vi "HFRR ADV v016 new software.vi"() -> ()   [LabVIEW 2025] (continued)
        n907 = call "IMAGE ANALYSIS.vi"("Enum"=POST_ANALYSIS_ENUM."SHOW UI", "error in"=w1070) -> ("error out"=w1068:errorcluster)  [unwired: 8 in, 1 out]
        n908 = local write "Zoom Factore"(100.0 ("Zoom Factore")) -> ()
      }
    }
    n909 = case shown="True" w759 {
      selector: w759 -> [_ w1047]
      tunnel: w751 -> [w1044 w1052]
      tunnel: [w1044 w1046] -> _
      frame False {
      }
      frame True {
        n910 = Not(x=w1047) -> (.not. x?=w1045:bool)
        n911 = local read "Zoom Factore"() -> (w1050:dbl)
        n912 = local write "OUT"(w1045) -> ()
        n913 = call "IMAGE ANALYSIS.vi"("Enum"=POST_ANALYSIS_ENUM."ZOOM OUT", "error in"=w1052) -> ("error out"=w1046:errorcluster)  [unwired: 8 in, 1 out]
        n914 = Divide(x=w1050, y=1.2) -> (x/y=w1048:dbl)
        n915 = local write "Zoom Factore"(w1048) -> ()
      }
    }
    n916 = case shown="True" w760 {
      selector: w760 -> [_ w1056]
      tunnel: w751 -> [w1053 w1061]
      tunnel: [w1053 w1054] -> _
      frame False {
      }
      frame True {
        n917 = Not(x=w1056) -> (.not. x?=w1055:bool)
        n918 = local read "Zoom Factore"() -> (w1059:dbl)
        n919 = local write "In"(w1055) -> ()
        n920 = call "IMAGE ANALYSIS.vi"("Enum"=POST_ANALYSIS_ENUM."ZOOM IN", "error in"=w1061) -> ("error out"=w1054:errorcluster)  [unwired: 8 in, 1 out]
        n921 = Multiply(x=w1059, y=1.2) -> (x*y=w1057:dbl)
        n922 = local write "Zoom Factore"(w1057) -> ()
      }
    }
    n923 = case shown="True" w756 {
      selector: w756 -> [_ w1028]
      tunnel: w751 -> [w1026 w1030]
      tunnel: [w1026 w1029] -> _
      frame False {
      }
      frame True {
        n924 = Not(x=w1028) -> (.not. x?=w1027:bool)
        n925 = local write "Clear ROI Tool"(w1027) -> ()
        n926 = call "IMAGE ANALYSIS.vi"("Enum"=POST_ANALYSIS_ENUM."CLEAR ROI", "error in"=w1030) -> ("error out"=w1029:errorcluster)  [unwired: 8 in, 1 out]
      }
    }
    n927 = case shown="True" w758 {
      selector: w758 -> [_ w1040]
      tunnel: w751 -> [w1038 w1043]
      tunnel: [w1038 w1041] -> _
      frame False {
      }
      frame True {
        n928 = Not(x=w1040) -> (.not. x?=w1039:bool)
        n929 = local write "line tool"(w1039) -> ()
        n930 = call "IMAGE ANALYSIS.vi"("Enum"=POST_ANALYSIS_ENUM."DRAW LINE", "error in"=w1043) -> ("error out"=w1041:errorcluster)  [unwired: 8 in, 1 out]
      }
    }
    n931 = case shown="True" w757 {
      selector: w757 -> [_ w1034]
      tunnel: w751 -> [w1032 w1036]
      tunnel: [w1032 w1035] -> _
      frame False {
      }
      frame True {
        n932 = Not(x=w1034) -> (.not. x?=w1033:bool)
        n933 = local write "Rectangle Tool"(w1033) -> ()
        n934 = call "IMAGE ANALYSIS.vi"("Enum"=POST_ANALYSIS_ENUM."DRAW REC", "error in"=w1036) -> ("error out"=w1035:errorcluster)  [unwired: 8 in, 1 out]
      }
    }
    n935 = local read "SCAR MEASURMENT"() -> (w744:enum32{"Auto Scar", "Manual Scar"})
    n936 = local read "Fit to Screen Tool"() -> (w753:bool)
    n937 = local read "Resize Tool"() -> (w752:bool)
    n938 = case shown="\"Manual Scar\", Default" w744 {
      frame "Auto Scar" {
        n939 = property on="Cap Live Image" class="Bool (strict)"("BoolText.Text"="Report" ("Boolean Text.Text")) -> ()  [unwired: 2 in, 2 out]
      }
      frame "Manual Scar", Default {
        n940 = property on="Cap Live Image" class="Bool (strict)"("BoolText.Text"="Save Image" ("Boolean Text.Text")) -> ()  [unwired: 2 in, 2 out]
      }
    }
    n941 = local read "ROI Color Tool"() -> (w754:bool)
    n942 = local read "Pan Tool"() -> (w755:bool)
    n943 = case shown="True" w755 {
      selector: w755 -> [_ w1022]
      tunnel: w751 -> [w1020 w1024]
      tunnel: [w1020 w1023] -> _
      frame False {
      }
      frame True {
        n944 = Not(x=w1022) -> (.not. x?=w1021:bool)
        n945 = call "IMAGE ANALYSIS.vi"("Enum"=POST_ANALYSIS_ENUM."PAN", "error in"=w1024) -> ("error out"=w1023:errorcluster)  [unwired: 8 in, 1 out]
        n946 = local write "Pan Tool"(w1021) -> ()
      }
    }
    n947 = case shown="True" w752 {
      selector: w752 -> [_ w1006]
      tunnel: w751 -> [w1001 w1003]
      tunnel: [w1001 w1002] -> _
      frame False {
      }
      frame True {
        n948 = Not(x=w1006) -> (.not. x?=w1005:bool)
        n949 = local write "Resize Tool"(w1005) -> ()
        n950 = call "IMAGE ANALYSIS.vi"("Enum"=POST_ANALYSIS_ENUM."RESIZE MODE", "error in"=w1003) -> ("error out"=w1002:errorcluster)  [unwired: 8 in, 1 out]
      }
    }
    n951 = case shown="True" w753 {
      selector: w753 -> [_ w1011]
      tunnel: [w1007 w1012] -> _
      tunnel: w751 -> [w1007 w1010]
      frame False {
      }
      frame True {
        n952 = Not(x=w1011) -> (.not. x?=w1009:bool)
        n953 = local write "Zoom Factore"(100.0 ("Zoom Factore")) -> ()
        n954 = local write "Fit to Screen Tool"(w1009) -> ()
        n955 = call "IMAGE ANALYSIS.vi"("Enum"=POST_ANALYSIS_ENUM."FIT", "error in"=w1010) -> ("error out"=w1012:errorcluster)  [unwired: 8 in, 1 out]
      }
    }
    n956 = case shown="True" w754 {
      selector: w754 -> [_ w1017]
      tunnel: [w1014 w1018] -> _
      tunnel: w751 -> [w1014 w1015]
      frame False {
      }
      frame True {
        n957 = Not(x=w1017) -> (.not. x?=w1016:bool)
        n958 = local write "ROI Color Tool"(w1016) -> ()
        n959 = call "IMAGE ANALYSIS.vi"("Enum"=POST_ANALYSIS_ENUM."SET ROI COLOR", "error in"=w1015) -> ("error out"=w1018:errorcluster)  [unwired: 8 in, 1 out]
      }
    }
    n960 = local read "Quit"() -> (w768:bool)
  }
  n961 = while {
    stop <- w1102 stop-if-true
    n962 = local read "Image Path"() -> (w1105:path)
    n963 = local read "Print 3"() -> (w1108:bool)
    n964 = Equal?(x=w1105, y=path "") -> (x = y?=w1104:bool)
    n965 = Not(x=w1104) -> (.not. x?=w1103:bool)
    n966 = property on="Print 3" class="Bool (strict)"("Visible"=w1103) -> ()  [unwired: 2 in, 2 out]
    n967 = case shown="True" w1108 {
      frame False {
        n968 = local write "Rd"(TRUE ("Boolean 7")) -> ()
      }
      frame True {
        n969 = flat-sequence {
          tunnel: [w1148] -> w1116
          tunnel: [w1135] -> w1114
          tunnel: [w1145] -> w1110
          tunnel: w1116 -> [w1157]
          tunnel: [w1157] -> w1115
          tunnel: w1114 -> [w1156]
          tunnel: [w1156] -> w1113
          tunnel: [w1154] -> w1112
          tunnel: [w1153] -> w1111
          tunnel: w1110 -> [w1153]
          tunnel: w1115 -> [w1159]
          tunnel: w1113 -> [w1160]
          tunnel: w1112 -> [_]
          tunnel: w1111 -> [w1158]
          frame #0 {
            n970 = case shown="True" "Rd" {
              frame False {
              }
              frame True {
                n971 = while {
                  tunnel: "abcdefABCDEF" ("string 2") -> [w1127]
                  shift-right: [w1125] -> w1119
                  shift-left: "" -> [w1124]
                  i -> [w1134]
                  stop <- w1133 stop-if-true
                  n972 = Random Number (0-1)() -> (number: 0 to 1=w1128:dbl)
                  n973 = Multiply(x=w1128, y=62.0) -> (x*y=w1130:dbl)
                  n974 = Decrement(x="Length 2") -> (x-1=w1123:i16)
                  n975 = To Word Integer(number=w1130) -> (16bit integer=w1131:i16)
                  n976 = String Subset(string=w1127, offset (0)=w1131, length (rest)=1 ("length (rest)")) -> (substring=w1126:string)
                  n977 = Greater Or Equal?(x=w1134, y=w1123) -> (x >= y?=w1133:bool)
                  n978 = Concatenate Strings(w1126, w1124) -> (w1125:string)
                }
                "String 10" <- w1119
                n979 = local write "Rd"(FALSE ("Boolean 7")) -> ()
              }
            }
          }
          frame #1 {
            w1146 = "_resized.jpg" ("command line")
            (unwired) ".jpg -resize 320x240 " ("string")
            (unwired) "Choose an Image File" ("prompt")
            # "-resize 1798x425"
            n980 = local read "Image Path"() -> (w1140:path)
            n981 = Strip Path(path=w1140) -> (stripped path=w1135:path, name=w1136:string)
            n982 = Match Pattern(string=w1136, regular expression=".jpg") -> (before substring=→"before substring 2":string, after substring=→"after substring":string)  [unwired: 1 in, 2 out]
            n983 = Match Pattern(string=w1136, regular expression="\\") -> (before substring=w1142:string)  [unwired: 1 in, 3 out]
            n984 = Match Pattern(string=w1142, regular expression=".jpg") -> (before substring=w1141:string)  [unwired: 1 in, 3 out]
            n985 = Concatenate Strings("cmd /c convert " ("string"), w1141, ".jpg -resize 320x240  " ("command line"), w1141, w1146) -> (w1149:string)
            n986 = call <vilib>:"System Exec.vi"("run minimized? (F)"=TRUE, "wait until completion? (T)"=TRUE, "working directory"=w1135, "command line"=w1149) -> ("error out"=w1148:errorcluster)  [unwired: 4 in, 3 out]
            "error out 2" <- w1148
            n987 = Concatenate Strings(w1141, w1146) -> (w1145:string)
          }
          frame #2 {
            n988 = Wait (ms)(milliseconds to wait=u32 2000 ("millisecond timer value")) -> (millisecond timer value=w1154:u32)
          }
          frame #3 {
            n989 = case shown="No Error" w1159 {
              tunnel: w1160 -> [w1163 _]
              tunnel: w1158 -> [w1161 _]
              frame No Error {
                (unwired) ".jpg" ("string")
                n990 = Path To String(path=w1163) -> (string=w1167:string)
                n991 = Concatenate Strings(w1167, "\\" ("string"), w1161) -> (w1166:string)
                n992 = String To Path(string=w1166) -> (path=w1165:path)
                n993 = call <vilib>:"Read JPEG File.vi"("path to JPEG file"=w1165) -> ("image data"=w1169:T16)  [unwired: 8 in, 2 out]
                "image data" <- w1169
                n994 = local write "Print 3"(FALSE ("Print 2")) -> ()
                n995 = call <vilib>:"Draw Flattened Pixmap.vi"("image data"=w1169) -> ("new picture"=→"new picture":picture)  [unwired: 8 in]
              }
              frame Error {
              }
            }
          }
        }
      }
    }
    n996 = Wait (ms)(milliseconds to wait=u32 20 ("millisecond timer value")) -> ()  [unwired: 1 out]
    n997 = local read "Quit"() -> (w1102:bool)
  }
  n998 = while {
    tunnel: w33 -> [_]
    tunnel: w17 -> [_]
    stop <- w1200 stop-if-true
    # "New Adv Logics"
    n999 = local read "Main Tab"() -> (w1180:T2)
    n1000 = local read "Main Tab"() -> (w1198:T2)
    n1001 = local read "Sign In"() -> (w1197:bool)
    n1002 = case shown="\"Adv Scar\"" w1180 {
      frame "HOME", Default {
        n1003 = local read "LIVE FEED MIN TEMP"() -> (w1333:bool)
        n1004 = local write "LIVE FEED MAX TEMP"(TRUE ("LIVE FEED MAX TEMP")) -> ()
        n1005 = local read "CAMERA ROI MIN TEMP"() -> (w1331:bool)
        n1006 = case shown="True" w1333 {
          selector: w1333 -> [_ w1340]
          frame False {
          }
          frame True {
            n1007 = Not(x=w1340) -> (.not. x?=w1339:bool)
            n1008 = local write "LIVE FEED MIN TEMP"(w1339) -> ()
            n1009 = call "CAMERA LIVE FEED FGV.vi"("Enum - Menu"=CAMERA_LIVE_FEED_ENUM."CAMERA MINIMIZE") -> ()  [unwired: 9 in, 2 out]
          }
        }
        n1010 = case shown="True" w1331 {
          selector: w1331 -> [_ w1337]
          frame False {
          }
          frame True {
            n1011 = Not(x=w1337) -> (.not. x?=w1336:bool)
            n1012 = local write "CAMERA ROI MIN TEMP"(w1336) -> ()
            n1013 = call "IMAGE ANALYSIS.vi"("Enum"=POST_ANALYSIS_ENUM."MINIMIZE UI") -> ()  [unwired: 9 in, 2 out]
          }
        }
        n1014 = local write "CAMERA ROI MAX TEMP"(TRUE ("CAMERA ROI MAX TEMP")) -> ()
      }
      frame "Test Setup" {
        n1015 = local read "LIVE FEED MIN TEMP"() -> (w1343:bool)
        n1016 = local read "CAMERA ROI MIN TEMP"() -> (w1341:bool)
        n1017 = local write "LIVE FEED MAX TEMP"(TRUE ("LIVE FEED MAX TEMP")) -> ()
        n1018 = case shown="True" w1343 {
          selector: w1343 -> [_ w1350]
          frame False {
          }
          frame True {
            n1019 = Not(x=w1350) -> (.not. x?=w1349:bool)
            n1020 = local write "LIVE FEED MIN TEMP"(w1349) -> ()
            n1021 = call "CAMERA LIVE FEED FGV.vi"("Enum - Menu"=CAMERA_LIVE_FEED_ENUM."CAMERA MINIMIZE") -> ()  [unwired: 9 in, 2 out]
          }
        }
        n1022 = case shown="True" w1341 {
          selector: w1341 -> [_ w1347]
          frame False {
          }
          frame True {
            n1023 = Not(x=w1347) -> (.not. x?=w1346:bool)
            n1024 = local write "CAMERA ROI MIN TEMP"(w1346) -> ()
            n1025 = call "IMAGE ANALYSIS.vi"("Enum"=POST_ANALYSIS_ENUM."MINIMIZE UI") -> ()  [unwired: 9 in, 2 out]
          }
        }
        n1026 = local write "CAMERA ROI MAX TEMP"(TRUE ("CAMERA ROI MAX TEMP")) -> ()
      }
      frame "Acquire" {
        n1027 = local read "LIVE FEED MIN TEMP"() -> (w1353:bool)
        n1028 = local write "LIVE FEED MAX TEMP"(TRUE ("LIVE FEED MAX TEMP")) -> ()
        n1029 = local read "CAMERA ROI MIN TEMP"() -> (w1351:bool)
        n1030 = case shown="True" w1353 {
          selector: w1353 -> [_ w1360]
          frame False {
          }
          frame True {
            n1031 = Not(x=w1360) -> (.not. x?=w1359:bool)
            n1032 = local write "LIVE FEED MIN TEMP"(w1359) -> ()
            n1033 = call "CAMERA LIVE FEED FGV.vi"("Enum - Menu"=CAMERA_LIVE_FEED_ENUM."CAMERA MINIMIZE") -> ()  [unwired: 9 in, 2 out]
          }
        }
        n1034 = case shown="True" w1351 {
          selector: w1351 -> [_ w1357]
          frame False {
          }
          frame True {
            n1035 = Not(x=w1357) -> (.not. x?=w1356:bool)
            n1036 = local write "CAMERA ROI MIN TEMP"(w1356) -> ()
            n1037 = call "IMAGE ANALYSIS.vi"("Enum"=POST_ANALYSIS_ENUM."MINIMIZE UI") -> ()  [unwired: 9 in, 2 out]
          }
        }
        n1038 = local write "CAMERA ROI MAX TEMP"(TRUE ("CAMERA ROI MAX TEMP")) -> ()
      }
      frame "Adv Scar" {
        n1039 = local read "CAMERA ROI MIN TEMP"() -> (w1361:bool)
        n1040 = case shown="True" "LIVE FEED MAX TEMP" {
          selector: "LIVE FEED MAX TEMP" -> [_ w1382]
          frame False {
          }
          frame True {
            n1041 = Not(x=w1382) -> (.not. x?=w1381:bool)
            n1042 = local write "LIVE FEED MAX TEMP"(w1381) -> ()
            n1043 = call "CAMERA LIVE FEED FGV.vi"("Enum - Menu"=CAMERA_LIVE_FEED_ENUM."CAMERA RESTORE") -> ("error out"=w1372:errorcluster)  [unwired: 9 in, 1 out]
            n1044 = Type Cast(type=30, x=0) -> (*(type *) &x=w1376:i32)
            n1045 = Add(x=w1376, y=48) -> (x+y=w1377:i32)
            n1046 = call "CAMERA LIVE FEED FGV.vi"("Enum - Menu"=CAMERA_LIVE_FEED_ENUM."CAMERA MODE SET", "error in (no error)"=w1372, "CAMERA MODE"=w1377) -> ("error out"=w1369:errorcluster)  [unwired: 7 in, 1 out]
            n1047 = call "CAMERA LIVE FEED FGV.vi"("Enum - Menu"=CAMERA_LIVE_FEED_ENUM."CAMERA GRAY", "error in (no error)"=w1369) -> ("error out"=w1368:errorcluster)  [unwired: 8 in, 1 out]
            n1048 = call "LIST FILE NAMES.vi"("error in (no error)"=w1368) -> ("error out"=w1378:errorcluster, "filenames"=w1379:string[])  [unwired: 9 in]
            n1049 = property on="FILE 3" class="CmbBox"(error in=w1378, "Strings[]"=w1379) -> ()  [unwired: 1 in, 2 out]
          }
        }
        n1050 = case shown="True" w1361 {
          selector: w1361 -> [_ w1367]
          frame False {
          }
          frame True {
            n1051 = Not(x=w1367) -> (.not. x?=w1366:bool)
            n1052 = local write "CAMERA ROI MIN TEMP"(w1366) -> ()
            n1053 = call "IMAGE ANALYSIS.vi"("Enum"=POST_ANALYSIS_ENUM."MINIMIZE UI") -> ()  [unwired: 9 in, 2 out]
          }
        }
        n1054 = local write "CAMERA ROI MAX TEMP"(TRUE ("CAMERA ROI MAX TEMP")) -> ()
        "LIVE FEED MIN TEMP" <- TRUE ("LIVE FEED MIN TEMP")
      }
      frame "Adv Scar Report" {
        n1055 = local read "CAMERA ROI MAX TEMP"() -> (w1383:bool)
        n1056 = local read "LIVE FEED MIN TEMP"() -> (w1385:bool)
        n1057 = local write "LIVE FEED MAX TEMP"(TRUE ("LIVE FEED MAX TEMP")) -> ()
        n1058 = case shown="True" w1385 {
          selector: w1385 -> [_ w1394]
          frame False {
          }
          frame True {
            n1059 = Not(x=w1394) -> (.not. x?=w1393:bool)
            n1060 = local write "LIVE FEED MIN TEMP"(w1393) -> ()
            n1061 = call "CAMERA LIVE FEED FGV.vi"("Enum - Menu"=CAMERA_LIVE_FEED_ENUM."CAMERA MINIMIZE") -> ()  [unwired: 9 in, 2 out]
          }
        }
        n1062 = case shown="True" w1383 {
          selector: w1383 -> [_ w1391]
          frame False {
          }
          frame True {
            n1063 = Not(x=w1391) -> (.not. x?=w1389:bool)
            n1064 = local write "CAMERA ROI MAX TEMP"(w1389) -> ()
            n1065 = call "IMAGE ANALYSIS.vi"("Enum"=POST_ANALYSIS_ENUM."SHOW UI") -> ("error out"=w1388:errorcluster)  [unwired: 9 in, 1 out]
            n1066 = call "LIST FILE NAMES.vi"("error in (no error)"=w1388) -> ("filenames"=w1387:string[])  [unwired: 9 in, 1 out]
            n1067 = property on="Test File List :" class="CmbBox"("Strings[]"=w1387) -> ()  [unwired: 2 in, 2 out]
          }
        }
        n1068 = local write "CAMERA ROI MIN TEMP"(TRUE ("CAMERA ROI MIN TEMP")) -> ()
      }
      frame "Compare Files" {
        n1069 = local read "LIVE FEED MIN TEMP"() -> (w1397:bool)
        n1070 = local write "LIVE FEED MAX TEMP"(TRUE ("LIVE FEED MAX TEMP")) -> ()
        n1071 = local read "CAMERA ROI MIN TEMP"() -> (w1395:bool)
        n1072 = case shown="True" w1397 {
          selector: w1397 -> [_ w1404]
          frame False {
          }
          frame True {
            n1073 = Not(x=w1404) -> (.not. x?=w1403:bool)
            n1074 = local write "LIVE FEED MIN TEMP"(w1403) -> ()
            n1075 = call "CAMERA LIVE FEED FGV.vi"("Enum - Menu"=CAMERA_LIVE_FEED_ENUM."CAMERA MINIMIZE") -> ()  [unwired: 9 in, 2 out]
          }
        }
        n1076 = case shown="True" w1395 {
          selector: w1395 -> [_ w1401]
          frame False {
          }
          frame True {
            n1077 = Not(x=w1401) -> (.not. x?=w1400:bool)
            n1078 = local write "CAMERA ROI MIN TEMP"(w1400) -> ()
            n1079 = call "IMAGE ANALYSIS.vi"("Enum"=POST_ANALYSIS_ENUM."MINIMIZE UI") -> ()  [unwired: 9 in, 2 out]
          }
        }
        n1080 = local write "CAMERA ROI MAX TEMP"(TRUE ("CAMERA ROI MAX TEMP")) -> ()
      }
      frame "About" {
        n1081 = local read "LIVE FEED MIN TEMP"() -> (w1407:bool)
        n1082 = local write "LIVE FEED MAX TEMP"(TRUE ("LIVE FEED MAX TEMP")) -> ()
        n1083 = local read "CAMERA ROI MIN TEMP"() -> (w1406:bool)
        n1084 = case shown="True" w1407 {
          selector: w1407 -> [_ w1414]
          frame False {
          }
          frame True {
            n1085 = Not(x=w1414) -> (.not. x?=w1413:bool)
            n1086 = local write "LIVE FEED MIN TEMP"(w1413) -> ()
            n1087 = call "CAMERA LIVE FEED FGV.vi"("Enum - Menu"=CAMERA_LIVE_FEED_ENUM."CAMERA MINIMIZE") -> ()  [unwired: 9 in, 2 out]
          }
        }
        n1088 = case shown="True" w1406 {
          selector: w1406 -> [_ w1411]
          frame False {
          }
          frame True {
            n1089 = Not(x=w1411) -> (.not. x?=w1410:bool)
            n1090 = local write "CAMERA ROI MIN TEMP"(w1410) -> ()
            n1091 = call "IMAGE ANALYSIS.vi"("Enum"=POST_ANALYSIS_ENUM."MINIMIZE UI") -> ()  [unwired: 9 in, 2 out]
          }
        }
        n1092 = local write "CAMERA ROI MAX TEMP"(TRUE ("CAMERA ROI MIN TEMP")) -> ()
      }
      frame "Advance" {
        n1093 = local read "LIVE FEED MIN TEMP"() -> (w1417:bool)
        n1094 = local write "LIVE FEED MAX TEMP"(TRUE ("LIVE FEED MAX TEMP")) -> ()
        n1095 = local read "CAMERA ROI MIN TEMP"() -> (w1415:bool)
        n1096 = case shown="True" w1417 {
          selector: w1417 -> [_ w1424]
          frame False {
          }
          frame True {
            n1097 = Not(x=w1424) -> (.not. x?=w1423:bool)
            n1098 = local write "LIVE FEED MIN TEMP"(w1423) -> ()
            n1099 = call "CAMERA LIVE FEED FGV.vi"("Enum - Menu"=CAMERA_LIVE_FEED_ENUM."CAMERA MINIMIZE") -> ()  [unwired: 9 in, 2 out]
          }
        }
        n1100 = local write "CAMERA ROI MAX TEMP"(TRUE ("CAMERA ROI MAX TEMP")) -> ()
        n1101 = case shown="True" w1415 {
          selector: w1415 -> [_ w1421]
          frame False {
          }
          frame True {
            n1102 = Not(x=w1421) -> (.not. x?=w1420:bool)
            n1103 = local write "CAMERA ROI MIN TEMP"(w1420) -> ()
            n1104 = call "IMAGE ANALYSIS.vi"("Enum"=POST_ANALYSIS_ENUM."MINIMIZE UI") -> ()  [unwired: 9 in, 2 out]
          }
        }
      }
      frame "Mooha" {
        n1105 = local read "LIVE FEED MIN TEMP"() -> (w1427:bool)
        n1106 = local write "LIVE FEED MAX TEMP"(TRUE ("LIVE FEED MAX TEMP")) -> ()
        n1107 = local read "CAMERA ROI MIN TEMP"() -> (w1425:bool)
        n1108 = case shown="True" w1427 {
          selector: w1427 -> [_ w1434]
          frame False {
          }
          frame True {
            n1109 = Not(x=w1434) -> (.not. x?=w1433:bool)
            n1110 = local write "LIVE FEED MIN TEMP"(w1433) -> ()
            n1111 = call "CAMERA LIVE FEED FGV.vi"("Enum - Menu"=CAMERA_LIVE_FEED_ENUM."CAMERA MINIMIZE") -> ()  [unwired: 9 in, 2 out]
          }
        }
        n1112 = local write "CAMERA ROI MAX TEMP"(TRUE ("CAMERA ROI MAX TEMP")) -> ()
        n1113 = case shown="True" w1425 {
          selector: w1425 -> [_ w1431]
          frame False {
          }
          frame True {
            n1114 = Not(x=w1431) -> (.not. x?=w1430:bool)
            n1115 = local write "CAMERA ROI MIN TEMP"(w1430) -> ()
            n1116 = call "IMAGE ANALYSIS.vi"("Enum"=POST_ANALYSIS_ENUM."MINIMIZE UI") -> ()  [unwired: 9 in, 2 out]
          }
        }
      }
    }
    n1117 = local read "Auto Start Test"() -> (w1171:bool)
    n1118 = case shown="True" "sign in temp" {
      frame False {
      }
      frame True {
        w1207 = 1 ("y")
        n1119 = local read "USERNAME"() -> (w1213:string)
        n1120 = local read "USER ID"() -> (w1210:string)
        n1121 = call <vilib>:"Trim Whitespace.vi"("string"=w1213) -> ("trimmed string"=w1212:string)  [unwired: 1 in]
        n1122 = call <vilib>:"Trim Whitespace.vi"("string"=w1210) -> ("trimmed string"=w1211:string)  [unwired: 1 in]
        n1123 = String Length(string=w1212) -> (length=w1209:i32)
        n1124 = String Length(string=w1211) -> (length=w1208:i32)
        n1125 = Greater?(x=w1209, y=w1207) -> (0:w1206:bool)
        n1126 = Greater?(x=w1208, y=w1207) -> (0:w1205:bool)
        n1127 = And(x=w1206, y=w1205) -> (x .and. y?=w1204:bool)
        n1128 = case shown="True" w1204 {
          frame False {
            n1129 = property on="Sign In" class="Bool (strict)"("DisabledEnum"=T18."Disabled" ("Disabled")) -> ()  [unwired: 2 in, 2 out]
          }
          frame True {
            n1130 = property on="Sign In" class="Bool (strict)"("DisabledEnum"=T18."Enabled" ("Disabled")) -> ()  [unwired: 2 in, 2 out]
          }
        }
      }
    }
    n1131 = local read "Air Temperature"() -> (w1188:bool)
    n1132 = local read "Coefficient Of Friction"() -> (w1189:bool)
    n1133 = case shown="False" w1171 {
      frame False {
        n1134 = local read "Auto stop temp"() -> (w1201:bool)
        n1135 = case shown="True" w1201 {
          frame False {
          }
          frame True {
            n1136 = local write "Auto Start Temp"(FALSE ("Auto Start Temp")) -> ()
          }
        }
      }
      frame True {
        "Auto stop temp" <- TRUE ("Auto stop temp")
      }
    }
    n1137 = local read "Humidity"() -> (w1187:bool)
    n1138 = case shown="\"HOME\"" w1198 {
      frame "HOME" {
        n1139 = local write "main tab sub"(enum32{"Page 1", "Page 2"}."Page 1" ("main tab sub")) -> ()
      }
      frame Default {
        n1140 = local write "main tab sub"(enum32{"Page 1", "Page 2"}."Page 2" ("main tab sub")) -> ()
      }
    }
    n1141 = case shown="True" w1197 {
      selector: w1197 -> [_ w1548]
      frame False {
      }
      frame True {
        n1142 = Not(x=w1548) -> (.not. x?=w1547:bool)
        n1143 = local write "Sign In"(w1547) -> ()
        n1144 = local write "Main Dashboard Buttons"(T24."Test Setup" ("Main Dashboard Buttons")) -> ()
      }
    }
    n1145 = case shown="\"Numeric Display\", Default" "Num/Graph" {
      frame "Numeric Display", Default {
        n1146 = property on="Single/Multiple" class="RadioBtnsControl (strict)"("Visible"=FALSE) -> ()  [unwired: 2 in, 2 out]
        n1147 = property on="Single - Graph" class="Ring (strict)"("Visible"=FALSE) -> ()  [unwired: 2 in, 2 out]
        n1148 = local write "Main Tab Display"(T4."Dashboard 1" ("Main Tab Display")) -> ()
      }
      frame "Graph Display" {
        n1149 = property on="Single/Multiple" class="RadioBtnsControl (strict)"("Visible"=TRUE) -> ()  [unwired: 2 in, 2 out]
        n1150 = case shown="\"Multiple\"" "Single/Multiple" {
          frame "Single ", Default {
            n1151 = property on="Single - Graph" class="Ring (strict)"("Visible"=TRUE) -> ()  [unwired: 2 in, 2 out]
            n1152 = local write "Main Tab Display"(T4."Dashboard 3" ("Main Tab Display")) -> ()
          }
          frame "Multiple" {
            n1153 = property on="Single - Graph" class="Ring (strict)"("Visible"=FALSE) -> ()  [unwired: 2 in, 2 out]
            n1154 = local write "Main Tab Display"(T4."Dashboard 2" ("Main Tab Display")) -> ()
          }
        }
      }
    }
    n1155 = local read "Stroke"() -> (w1186:bool)
    n1156 = local read "USERNAME"() -> (w1192:string)
    n1157 = local read "USER ID"() -> (w1191:string)
    n1158 = case shown="True" w1189 {
      selector: w1189 -> [_ w1474]
      frame False {
      }
      frame True {
        n1159 = Not(x=w1474) -> (.not. x?=w1473:bool)
        n1160 = local write "Coefficient Of Friction"(w1473) -> ()
        n1161 = local write "Tab Control 2"(T6."Coefficient Of Friction" ("Tab Control 2")) -> ()
      }
    }
    n1162 = case shown="True" w1188 {
      selector: w1188 -> [_ w1471]
      frame False {
      }
      frame True {
        n1163 = Not(x=w1471) -> (.not. x?=w1469:bool)
        n1164 = local write "Air Temperature"(w1469) -> ()
        n1165 = local write "Tab Control 2"(T6."Air Temperature" ("Tab Control 2")) -> ()
      }
    }
    n1166 = local write "Operator ID"(w1191) -> ()
    n1167 = case shown="True" w1186 {
      selector: w1186 -> [_ w1465]
      frame False {
      }
      frame True {
        n1168 = Not(x=w1465) -> (.not. x?=w1463:bool)
        n1169 = local write "Stroke"(w1463) -> ()
        n1170 = local write "Tab Control 2"(T6."Stroke" ("Tab Control 2")) -> ()
      }
    }
    n1171 = local write "tested by"(w1192) -> ()
    n1172 = case shown="True" w1187 {
      selector: w1187 -> [_ w1468]
      frame False {
      }
      frame True {
        n1173 = Not(x=w1468) -> (.not. x?=w1466:bool)
        n1174 = local write "Humidity"(w1466) -> ()
        n1175 = local write "Tab Control 2"(T6."Humidity" ("Tab Control 2")) -> ()
      }
    }
    n1176 = case shown="\"Calibration\"" "Main Dashboard Buttons" {
      tunnel: [T2."HOME" ("Main Tab") T2."Test Setup" ("Main Tab") T2."Acquire" ("Main Tab") T2."Adv Scar" ("Main Tab") T2."Adv Scar Report" ("Main Tab") T2."Compare Files" ("Main Tab") T2."Calibration" ("Main Tab") T2."About" ("Main Tab") T2."Advance" ("Main Tab")] -> w1170
      frame "Home", Default {
      }
      frame "Test Setup" {
      }
      frame "Dashboard" {
      }
      frame "Imaging" {
      }
      frame "Report" {
      }
      frame "Analysis" {
      }
      frame "Calibration" {
      }
      frame "About" {
      }
      frame "Advance" {
      }
    }
    n1177 = Wait (ms)(milliseconds to wait=u32 100) -> ()  [unwired: 1 out]
    n1178 = local read "Main Tab Display"() -> (w1190:T4)
    n1179 = local write "Main Tab"(w1170) -> ()
    n1180 = case shown="\"Dashboard 3\"" w1190 {
      frame "Dashboard 1", Default {
        n1181 = property on="Reset Graph" class="Bool (strict)"("Visible"=FALSE) -> ()  [unwired: 2 in, 2 out]
      }
      frame "Dashboard 2" {
        n1182 = property on="Reset Graph" class="Bool (strict)"("Visible"=TRUE) -> ()  [unwired: 2 in, 2 out]
      }
      frame "Dashboard 3" {
        n1183 = property on="Reset Graph" class="Bool (strict)"("Visible"=TRUE) -> ()  [unwired: 2 in, 2 out]
      }
    }
    n1184 = local read "SCAR MEASURMENT"() -> (w1178:enum32{"Auto Scar", "Manual Scar"})
    n1185 = local read "Humidity"() -> (w1193:bool)
    n1186 = local read "Cap Live Image"() -> (w1175:bool)
    n1187 = local read "Sample Temperature"() -> (w1185:bool)
    n1188 = local read "Air Temp vs Humidity"() -> (w1183:bool)
    n1189 = local read "Frequency"() -> (w1184:bool)
    n1190 = case shown="True" w1193 {
      frame False {
        n1191 = local write "Humidity On Command"(TRUE ("Humidity On Command")) -> ()
        n1192 = case shown="True" "Humidity Off Command" {
          selector: "Humidity Off Command" -> [_ w1481]
          frame False {
          }
          frame True {
            n1193 = stacked-sequence {
              frame #0 {
                n1194 = local read "WriteHumidity"() -> (w1483:string[])
                n1195 = Insert Into Array(array=w1483, new element="R;1" ("new element/subarray")) -> (w1484:string[])  [unwired: 1 in]
                n1196 = local write "WriteHumidity"(w1484) -> ()
              }
              frame #1 {
                n1197 = Wait (ms)(milliseconds to wait=u32 2000) -> ()  [unwired: 1 out]
              }
              frame #2 {
                n1198 = local read "EVENT LOG"() -> (w1490:string)
                n1199 = local read "WriteHumidity"() -> (w1487:string[])
                n1200 = call "Event Log.vi"("Content"="Humidity Control Off" ("string"), "EVENT LOG"=w1490) -> ("EVENT LOG"=w1491:string)  [unwired: 8 in, 1 out]
                n1201 = local write "EVENT LOG"(w1491) -> ()
                n1202 = Insert Into Array(array=w1487, new element="R;1" ("new element/subarray")) -> (w1488:string[])  [unwired: 1 in]
                n1203 = local write "WriteHumidity"(w1488) -> ()
              }
            }
            n1204 = Not(x=w1481) -> (.not. x?=w1480:bool)
            n1205 = local write "Humidity Off Command"(w1480) -> ()
          }
        }
      }
      frame True {
        n1206 = local write "Humidity Off Command"(TRUE ("Humidity Off Command")) -> ()
        n1207 = case shown="True" "Humidity On Command" {
          selector: "Humidity On Command" -> [_ w1495]
          frame False {
          }
          frame True {
            n1208 = stacked-sequence {
              frame #0 {
                n1209 = local read "Set Rh"() -> (w1501:dbl)
                n1210 = Number To Fractional String(number=w1501, precision (6)=i16 2) -> (F-format string=w1502:string)  [unwired: 2 in]
                n1211 = local read "WriteHumidity"() -> (w1499:string[])
                n1212 = Concatenate Strings("M;" ("new element/subarray"), w1502) -> (w1500:string)
                n1213 = Insert Into Array(array=w1499, new element=w1500) -> (w1498:string[])  [unwired: 1 in]
                n1214 = local write "WriteHumidity"(w1498) -> ()
              }
              frame #1 {
                n1215 = Wait (ms)(milliseconds to wait=u32 2000) -> ()  [unwired: 1 out]
              }
              frame #2 {
                n1216 = local read "Set Rh"() -> (w1509:dbl)
                n1217 = Number To Fractional String(number=w1509, precision (6)=i16 2) -> (F-format string=w1510:string)  [unwired: 2 in]
                n1218 = local read "WriteHumidity"() -> (w1507:string[])
                n1219 = Concatenate Strings("M;" ("new element/subarray"), w1510) -> (w1508:string)
                n1220 = Insert Into Array(array=w1507, new element=w1508) -> (w1506:string[])  [unwired: 1 in]
                n1221 = local write "WriteHumidity"(w1506) -> ()
              }
              frame #3 {
                n1222 = Wait (ms)(milliseconds to wait=u32 1500) -> ()  [unwired: 1 out]
              }
              frame #4 {
                (unwired) "% RH" ("string")
                (unwired) i16 2 ("precision (6)")
                (unwired) "M;" ("new element/subarray")
                n1223 = local read "Set Rh"() -> (w1517:dbl)
                n1224 = Number To Fractional String(number=w1517, precision (6)=i16 2) -> (F-format string=w1514:string)  [unwired: 2 in]
                n1225 = local read "WriteHumidity"() -> (w1519:string[])
                n1226 = Concatenate Strings("M;" ("new element/subarray"), w1514) -> (w1518:string)
                n1227 = Concatenate Strings("Humidity Set to : " ("string"), w1514, "% RH" ("string")) -> (w1512:string)
                n1228 = Insert Into Array(array=w1519, new element=w1518) -> (w1520:string[])  [unwired: 1 in]
                n1229 = disable-structure shown="Enabled" {
                  frame Enabled {
                    n1230 = local read "EVENT LOG"() -> (w1523:string)
                    n1231 = call "Event Log.vi"("Content"="Humidity Control On", "EVENT LOG"=w1523) -> ("EVENT LOG"=w1524:string)  [unwired: 8 in, 1 out]
                    n1232 = local write "EVENT LOG"(w1524) -> ()
                  }
                  frame Disabled {
                  }
                }
                n1233 = disable-structure shown="Enabled" {
                  disable-tunnel: w1512 -> [_ _]
                  frame Enabled {
                    n1234 = local read "EVENT LOG"() -> (w1526:string)
                    n1235 = call "Event Log.vi"("Content"="Humidity Control On", "EVENT LOG"=w1526) -> ("EVENT LOG"=w1527:string)  [unwired: 8 in, 1 out]
                    n1236 = local write "EVENT LOG"(w1527) -> ()
                  }
                  frame Disabled {
                  }
                }
                n1237 = local write "WriteHumidity"(w1520) -> ()
              }
            }
            n1238 = Not(x=w1495) -> (.not. x?=w1494:bool)
            n1239 = local write "Humidity On Command"(w1494) -> ()
          }
        }
      }
    }
    n1240 = Equal?(x=w1178, y=enum32{"Auto Scar", "Manual Scar"}."Auto Scar" ("SCAR MEASURMENT")) -> (x = y?=w1174:bool)
    n1241 = local read "TEST STANDARD"() -> (w1181:T3)
    n1242 = And(x=w1175, y=w1174) -> (x .and. y?=w1176:bool)
    n1243 = case shown="True" w1176 {
      selector: w1176 -> [_ w1280]
      tunnel: errorcluster {"status"=FALSE, "code"=0, "source"=""} ("error in (no error) 3") -> [_ w1281]
      frame False {
      }
      frame True {
        n1244 = stacked-sequence {
          tunnel: w1281 -> [_ _ _ _ _ _ _ w1329]
          tunnel: w1280 -> [_ _ _ _ _ w1310 _ _]
          frame #0 {
            n1245 = call "CAMERA LIVE FEED FGV.vi"("Enum - Menu"=CAMERA_LIVE_FEED_ENUM."CAMERA MINIMIZE") -> ()  [unwired: 9 in, 2 out]
          }
          frame #1 {
            n1246 = property on="Auto Scar Check  2" class="Clust (strict)"("Visible"=TRUE) -> ()  [unwired: 2 in, 2 out]
          }
          frame #2 {
            n1247 = String To Path(string="C:\\LAB-IQ\\Image Calibrate v01.dcf") -> (path=w1286:path)
            n1248 = Open/Create/Replace File ("Open File")(file path (use dialog)=w1286) -> (refnum out=w1287:refnum<file>)  [unwired: 5 in, 2 out]
            n1249 = for {
              N: 4 -> [_]
              tunnel: w1287 -> [w1293]
              i -> [w1289]
              n1250 = Read from Text File ("Read File")(file (use dialog)=w1293) -> (text=w1294:string)  [unwired: 3 in, 3 out]
              n1251 = String Subset(string=w1294, offset (0)=6, length (rest)=10 ("length (rest)")) -> (substring=w1290:string)
              n1252 = Fract/Exp String To Number(string=w1290) -> (number=w1288:dbl)  [unwired: 3 in, 1 out]
              n1253 = case shown="0" w1289 {
                tunnel: w1288 -> [w1295 w1296 _ w1297 _]
                frame 0 {
                  "5x Gain" <- w1295
                }
                frame 1 {
                  "10x Gain" <- w1296
                }
                frame 2 {
                }
                frame 3 {
                  "100x gain" <- w1297
                }
                frame 4, Default {
                }
              }
            }
          }
          frame #3 {
            n1254 = local read "FILE 3"() -> (w1303:string)
            n1255 = call <vilib>:"Trim Whitespace.vi"("string"="C:\\LAB-IQ\\images\\") -> ("trimmed string"=w1305:string)  [unwired: 1 in]
            n1256 = String To Path(string=w1305) -> (path=w1304:path)
            n1257 = Concatenate Strings(w1303, ".png" ("string")) -> (w1302:string)
            n1258 = Build Path(base path=w1304, name or relative path=w1302) -> (appended path=w1300:path)
            "Image path" <- w1300
            n1259 = Path To String(path=w1300) -> (string=w1299:string)
            n1260 = call "CAMERA LIVE FEED FGV.vi"("Enum - Menu"=CAMERA_LIVE_FEED_ENUM."CAMERA SAVE", "Image Path"=w1299) -> ()  [unwired: 8 in, 2 out]
          }
          frame #4 {
            n1261 = One Button Dialog(message="Image saved successfully") -> ()  [unwired: 1 in, 1 out]
          }
          frame #5 {
            n1262 = local read "TEST STANDARD"() -> (w1309:T3)
            n1263 = local read "Magnification len live scar"() -> (w1321:string)
            n1264 = Not(x=w1310) -> (.not. x?=w1311:bool)
            n1265 = local write "Cap Live Image"(w1311) -> ()
            n1266 = case shown="\"ISO 12156\"" w1309 {
              tunnel: ["ASTM D6079" "ISO 12156"] -> w1308
              frame "ASTM D6079", Default {
              }
              frame "ISO 12156" {
              }
            }
            n1267 = case shown="\"5x\", Default" w1321 {
              tunnel: [w1324 w1325] -> w1320
              frame "5x", Default {
                n1268 = local read "5x Gain"() -> (w1324:dbl)
              }
              frame "10x" {
                # "5x"
                n1269 = local read "10x Gain"() -> (w1325:dbl)
              }
            }
            n1270 = local read "Image path"() -> (w1319:path)
            n1271 = local read "FILE 3"() -> (w1312:string)
            n1272 = call "EDGE DETCTION.vi"("GAIN VALUE"=w1320, "Image Path"=w1319) -> ("error out"=w1318:errorcluster, "return value"=w1317:cluster{string, string, dbl, dbl, dbl})  [unwired: 8 in]
            n1273 = Bundle By Name(cluster=T25 {"File Name"="", "Test Method"="", "Operator"="", "Fuel Description"="", "Date and time"=""} ("Main Ref"), "File Name"=w1312, "Test Method"=w1308) -> (w1313:T25)
            n1274 = call "duf file read.vi"("error in (no error)"=w1318, "Main Ref"=w1313) -> ("error out"=w1316:errorcluster, "Main Ref 2"=w1314:T25)  [unwired: 8 in]
            n1275 = call "EDGE DETECTION REPORT.vi"("error in (no error)"=w1316, "return value 2"=w1317, "Main Ref"=w1314) -> ()  [unwired: 8 in, 1 out]
          }
          frame #6 {
            n1276 = property on="Auto Scar Check  2" class="Clust (strict)"("Visible"=FALSE) -> ()  [unwired: 2 in, 2 out]
          }
          frame #7 {
            n1277 = call "CAMERA LIVE FEED FGV.vi"("Enum - Menu"=CAMERA_LIVE_FEED_ENUM."CAMERA MINIMIZE", "error in (no error)"=w1329) -> ()  [unwired: 8 in, 2 out]
            n1278 = local write "Main Dashboard Buttons"(T1."Home" ("Main Dashboard Buttons")) -> ()
            n1279 = local write "Main Tab"(T2."HOME" ("Main Tab")) -> ()
          }
        }
      }
    }
    n1280 = local read "Heater Button"() -> (w1182:bool)
    n1281 = case shown="True" w1184 {
      selector: w1184 -> [_ w1459]
      frame False {
      }
      frame True {
        n1282 = Not(x=w1459) -> (.not. x?=w1457:bool)
        n1283 = local write "Frequency"(w1457) -> ()
        n1284 = local write "Tab Control 2"(T6."Frequency" ("Tab Control 2")) -> ()
      }
    }
    n1285 = case shown="True" w1183 {
      selector: w1183 -> [_ w1456]
      frame False {
      }
      frame True {
        n1286 = Not(x=w1456) -> (.not. x?=w1454:bool)
        n1287 = local write "Air Temp vs Humidity"(w1454) -> ()
        n1288 = local write "Tab Control 2"(T6."Air Temp vs Rh" ("Tab Control 2")) -> ()
      }
    }
    n1289 = case shown="True" w1185 {
      selector: w1185 -> [_ w1462]
      frame False {
      }
      frame True {
        n1290 = Not(x=w1462) -> (.not. x?=w1460:bool)
        n1291 = local write "Sample Temperature"(w1460) -> ()
        n1292 = local write "Tab Control 2"(T6."Sample Temperature" ("Tab Control 2")) -> ()
      }
    }
    n1293 = case shown="\"Custom\"" w1181 {
      frame "ASTM D6079", Default {
        w1435 = "ASTM D6079 TEST CONDITIONS" ("Standard 2")
        n1294 = local write "Standard 2"(w1435) -> ()
        n1295 = local write "Standard"(w1435) -> ()
      }
      frame "ISO 12156" {
        w1436 = "ISO 12156 TEST CONDITIONS" ("Standard 2")
        n1296 = local write "Standard 2"(w1436) -> ()
        n1297 = local write "Standard"(w1436) -> ()
      }
      frame "CEC F-096-A-06" {
        w1437 = "CEC F-096-A-06 TEST CONDITIONS" ("Standard 2")
        n1298 = local write "Standard 2"(w1437) -> ()
        n1299 = local write "Standard"(w1437) -> ()
      }
      frame "Custom" {
        w1438 = "CUSTOM TEST CONDITIONS" ("Standard 2")
        n1300 = local write "Standard 2"(w1438) -> ()
        n1301 = local write "Standard"(w1438) -> ()
      }
    }
    n1302 = case shown="True" w1182 {
      frame False {
        n1303 = local write "Temperature On Command"(TRUE ("Temperature On Command")) -> ()
        n1304 = case shown="True" "Temperature Off Command" {
          selector: "Temperature Off Command" -> [_ w1442]
          frame False {
          }
          frame True {
            n1305 = Not(x=w1442) -> (.not. x?=w1441:bool)
            n1306 = local read "EVENT LOG"() -> (w1445:string)
            n1307 = local write "Temperature Off Command"(w1441) -> ()
            n1308 = call "Event Log.vi"("Content"="Heater Off", "EVENT LOG"=w1445) -> ("EVENT LOG"=w1444:string)  [unwired: 8 in, 1 out]
            n1309 = local write "EVENT LOG"(w1444) -> ()
          }
        }
      }
      frame True {
        n1310 = local write "Temperature Off Command"(TRUE ("Temperature Off Command")) -> ()
        n1311 = case shown="True" "Temperature On Command" {
          selector: "Temperature On Command" -> [_ w1449]
          frame False {
          }
          frame True {
            n1312 = Not(x=w1449) -> (.not. x?=w1448:bool)
            n1313 = local write "Temperature On Command"(w1448) -> ()
            n1314 = disable-structure shown="Enabled" {
              disable-tunnel: "Heater On" -> [w1451 _]
              frame Enabled {
                n1315 = local read "EVENT LOG"() -> (w1452:string)
                n1316 = call "Event Log.vi"("Content"=w1451, "EVENT LOG"=w1452) -> ("EVENT LOG"=w1453:string)  [unwired: 8 in, 1 out]
                n1317 = local write "EVENT LOG"(w1453) -> ()
              }
              frame Disabled {
              }
            }
          }
        }
      }
    }
    n1318 = local read "Main Tab"() -> (w1173:T2)
    n1319 = case shown="\"About\"" w1173 {
      frame "HOME", Default {
        w1216 = T18."Enabled" ("Disabled")
        n1320 = local read "Service Password enable"() -> (w1218:bool)
        n1321 = property on="Imaging" class="Bool (strict)"("DisabledEnum"=w1216) -> ()  [unwired: 2 in, 2 out]
        n1322 = property on="Dashboard" class="Bool (strict)"("DisabledEnum"=w1216) -> ()  [unwired: 2 in, 2 out]
        n1323 = property on="Test Setup" class="Bool (strict)"("DisabledEnum"=w1216) -> ()  [unwired: 2 in, 2 out]
        n1324 = property on="Analysis" class="Bool (strict)"("DisabledEnum"=w1216) -> ()  [unwired: 2 in, 2 out]
        n1325 = property on="Home" class="Bool (strict)"("DisabledEnum"=w1216) -> ()  [unwired: 2 in, 2 out]
        n1326 = property on="Report" class="Bool (strict)"("DisabledEnum"=w1216) -> ()  [unwired: 2 in, 2 out]
        n1327 = property on="Main Dashboard Buttons" class="RadioBtnsControl (strict)"("DisabledEnum"=w1216) -> ()  [unwired: 2 in, 2 out]
        n1328 = property on="Calibration" class="Bool (strict)"("DisabledEnum"=w1216) -> ()  [unwired: 2 in, 2 out]
        n1329 = case shown="True" w1218 {
          tunnel: [T18."Disabled" ("Disabled") T18."Enabled" ("Disabled")] -> w1217
          frame False {
          }
          frame True {
          }
        }
        n1330 = property on="About" class="Bool (strict)"("DisabledEnum"=w1217) -> ()  [unwired: 2 in, 2 out]
      }
      frame "Test Setup" {
        w1223 = T18."Enabled" ("Disabled")
        n1331 = local read "Service Password enable"() -> (w1222:bool)
        n1332 = property on="Dashboard" class="Bool (strict)"("DisabledEnum"=T18."Disabled" ("Disabled")) -> ()  [unwired: 2 in, 2 out]
        n1333 = property on="Imaging" class="Bool (strict)"("DisabledEnum"=w1223) -> ()  [unwired: 2 in, 2 out]
        n1334 = property on="Analysis" class="Bool (strict)"("DisabledEnum"=w1223) -> ()  [unwired: 2 in, 2 out]
        n1335 = property on="Home" class="Bool (strict)"("DisabledEnum"=w1223) -> ()  [unwired: 2 in, 2 out]
        n1336 = property on="Report" class="Bool (strict)"("DisabledEnum"=w1223) -> ()  [unwired: 2 in, 2 out]
        n1337 = property on="Test Setup" class="Bool (strict)"("DisabledEnum"=w1223) -> ()  [unwired: 2 in, 2 out]
        n1338 = case shown="True" w1222 {
          tunnel: [T18."Disabled" ("Disabled") T18."Enabled" ("Disabled")] -> w1221
          frame False {
          }
          frame True {
          }
        }
        n1339 = property on="About" class="Bool (strict)"("DisabledEnum"=w1221) -> ()  [unwired: 2 in, 2 out]
      }
      frame "Adv Scar" {
        w1230 = T18."Enabled" ("Disabled")
        n1340 = property on="Dashboard" class="Bool (strict)"("DisabledEnum"=T18."Disabled" ("Disabled")) -> ()  [unwired: 2 in, 2 out]
        n1341 = property on="Imaging" class="Bool (strict)"("DisabledEnum"=w1230) -> ()  [unwired: 2 in, 2 out]
        n1342 = property on="Analysis" class="Bool (strict)"("DisabledEnum"=w1230) -> ()  [unwired: 2 in, 2 out]
        n1343 = property on="Home" class="Bool (strict)"("DisabledEnum"=w1230) -> ()  [unwired: 2 in, 2 out]
        n1344 = property on="Report" class="Bool (strict)"("DisabledEnum"=w1230) -> ()  [unwired: 2 in, 2 out]
        n1345 = property on="Test Setup" class="Bool (strict)"("DisabledEnum"=w1230) -> ()  [unwired: 2 in, 2 out]
        n1346 = local read "Service Password enable"() -> (w1228:bool)
        n1347 = case shown="True" w1228 {
          tunnel: [T18."Disabled" ("Disabled") T18."Enabled" ("Disabled")] -> w1227
          frame False {
          }
          frame True {
          }
        }
        n1348 = property on="About" class="Bool (strict)"("DisabledEnum"=w1227) -> ()  [unwired: 2 in, 2 out]
      }
      frame "Calibration" {
        w1233 = T18."Enabled" ("Disabled")
        n1349 = property on="Dashboard" class="Bool (strict)"("DisabledEnum"=T18."Disabled" ("Disabled")) -> ()  [unwired: 2 in, 2 out]
        n1350 = property on="Imaging" class="Bool (strict)"("DisabledEnum"=w1233) -> ()  [unwired: 2 in, 2 out]
        n1351 = property on="Analysis" class="Bool (strict)"("DisabledEnum"=w1233) -> ()  [unwired: 2 in, 2 out]
        n1352 = property on="Home" class="Bool (strict)"("DisabledEnum"=w1233) -> ()  [unwired: 2 in, 2 out]
        n1353 = property on="Report" class="Bool (strict)"("DisabledEnum"=w1233) -> ()  [unwired: 2 in, 2 out]
        n1354 = property on="Test Setup" class="Bool (strict)"("DisabledEnum"=w1233) -> ()  [unwired: 2 in, 2 out]
        n1355 = local read "Service Password enable"() -> (w1235:bool)
        n1356 = property on="Calibration" class="Bool (strict)"("DisabledEnum"=w1233) -> ()  [unwired: 2 in, 2 out]
        n1357 = case shown="True" w1235 {
          tunnel: [T18."Disabled" ("Disabled") T18."Enabled" ("Disabled")] -> w1234
          frame False {
          }
          frame True {
          }
        }
        n1358 = property on="About" class="Bool (strict)"("DisabledEnum"=w1234) -> ()  [unwired: 2 in, 2 out]
      }
      frame "Adv Scar Report" {
        w1241 = T18."Enabled" ("Disabled")
        n1359 = property on="Dashboard" class="Bool (strict)"("DisabledEnum"=T18."Disabled" ("Disabled")) -> ()  [unwired: 2 in, 2 out]
        n1360 = property on="Imaging" class="Bool (strict)"("DisabledEnum"=w1241) -> ()  [unwired: 2 in, 2 out]
        n1361 = property on="Analysis" class="Bool (strict)"("DisabledEnum"=w1241) -> ()  [unwired: 2 in, 2 out]
        n1362 = property on="Home" class="Bool (strict)"("DisabledEnum"=w1241) -> ()  [unwired: 2 in, 2 out]
        n1363 = property on="Report" class="Bool (strict)"("DisabledEnum"=w1241) -> ()  [unwired: 2 in, 2 out]
        n1364 = property on="Test Setup" class="Bool (strict)"("DisabledEnum"=w1241) -> ()  [unwired: 2 in, 2 out]
        n1365 = local read "Service Password enable"() -> (w1240:bool)
        n1366 = case shown="True" w1240 {
          tunnel: [T18."Disabled" ("Disabled") T18."Enabled" ("Disabled")] -> w1239
          frame False {
          }
          frame True {
          }
        }
        n1367 = property on="About" class="Bool (strict)"("DisabledEnum"=w1239) -> ()  [unwired: 2 in, 2 out]
      }
      frame "Compare Files" {
        w1247 = T18."Enabled" ("Disabled")
        n1368 = local read "Service Password enable"() -> (w1246:bool)
        n1369 = property on="Dashboard" class="Bool (strict)"("DisabledEnum"=T18."Disabled" ("Disabled")) -> ()  [unwired: 2 in, 2 out]
        n1370 = property on="Imaging" class="Bool (strict)"("DisabledEnum"=w1247) -> ()  [unwired: 2 in, 2 out]
        n1371 = property on="Analysis" class="Bool (strict)"("DisabledEnum"=w1247) -> ()  [unwired: 2 in, 2 out]
        n1372 = property on="Home" class="Bool (strict)"("DisabledEnum"=w1247) -> ()  [unwired: 2 in, 2 out]
        n1373 = property on="Report" class="Bool (strict)"("DisabledEnum"=w1247) -> ()  [unwired: 2 in, 2 out]
        n1374 = property on="Test Setup" class="Bool (strict)"("DisabledEnum"=w1247) -> ()  [unwired: 2 in, 2 out]
        n1375 = case shown="True" w1246 {
          tunnel: [T18."Disabled" ("Disabled") T18."Enabled" ("Disabled")] -> w1245
          frame False {
          }
          frame True {
          }
        }
        n1376 = property on="About" class="Bool (strict)"("DisabledEnum"=w1245) -> ()  [unwired: 2 in, 2 out]
      }
      frame "Acquire" {
        n1377 = local read "Service Password enable"() -> (w1252:bool)
        n1378 = property on="Test Setup" class="Bool (strict)"("DisabledEnum"=T18."Disabled" ("Disabled")) -> ()  [unwired: 2 in, 2 out]
        n1379 = local read "Auto Start Test"() -> (w1254:bool)
        n1380 = local read "RUN"() -> (w1256:bool)
        n1381 = case shown="True" w1252 {
          tunnel: [T18."Disabled" ("Disabled") T18."Enabled" ("Disabled")] -> w1253
          frame False {
          }
          frame True {
          }
        }
        n1382 = Or(x=w1256, y=w1254) -> (x .or. y?=w1255:bool)
        n1383 = case shown="True" w1255 {
          tunnel: [T18."Enabled" ("Disabled") T18."Disabled" ("Disabled")] -> w1251
          frame False {
          }
          frame True {
          }
        }
        n1384 = property on="About" class="Bool (strict)"("DisabledEnum"=w1253) -> ()  [unwired: 2 in, 2 out]
        n1385 = property on="Imaging" class="Bool (strict)"("DisabledEnum"=w1251) -> ()  [unwired: 2 in, 2 out]
        n1386 = property on="Dashboard" class="Bool (strict)"("DisabledEnum"=w1251) -> ()  [unwired: 2 in, 2 out]
        n1387 = property on="Analysis" class="Bool (strict)"("DisabledEnum"=w1251) -> ()  [unwired: 2 in, 2 out]
        n1388 = property on="Home" class="Bool (strict)"("DisabledEnum"=w1251) -> ()  [unwired: 2 in, 2 out]
        n1389 = property on="Report" class="Bool (strict)"("DisabledEnum"=w1251) -> ()  [unwired: 2 in, 2 out]
        n1390 = property on="Calibration" class="Bool (strict)"("DisabledEnum"=w1251) -> ()  [unwired: 2 in, 2 out]
      }
      frame "About" {
        n1391 = local read "FILE"() -> (w1270:string)
        n1392 = local read "TEST FILE NAM,E SAVED"() -> (w1263:bool)
        n1393 = call <vilib>:"Trim Whitespace.vi"("string"=w1270) -> ("trimmed string"=w1269:string)  [unwired: 1 in]
        n1394 = local read "Auto Start Test"() -> (w1273:bool)
        n1395 = String Length(string=w1269) -> (length=w1268:i32)
        n1396 = Greater?(x=w1268, y=1) -> (0:w1265:bool)
        n1397 = And(x=w1265, y=w1263) -> (x .and. y?=w1264:bool)
        n1398 = local read "RUN"() -> (w1275:bool)
        n1399 = case shown="True" w1264 {
          tunnel: [T18."Disabled" ("Disabled") T18."Enabled" ("Disabled")] -> w1266
          frame False {
          }
          frame True {
          }
        }
        n1400 = Or(x=w1275, y=w1273) -> (x .or. y?=w1274:bool)
        n1401 = property on="About" class="Bool (strict)"("DisabledEnum"=T18."Enabled" ("Disabled")) -> ()  [unwired: 2 in, 2 out]
        n1402 = case shown="False" w1274 {
          tunnel: [T18."Enabled" ("Disabled") T18."Disabled" ("Disabled")] -> w1272
          frame False {
          }
          frame True {
          }
        }
        n1403 = property on="Dashboard" class="Bool (strict)"("DisabledEnum"=w1266) -> ()  [unwired: 2 in, 2 out]
        n1404 = property on="Test Setup" class="Bool (strict)"("DisabledEnum"=T18."Disabled" ("Disabled")) -> ()  [unwired: 2 in, 2 out]
        n1405 = property on="Imaging" class="Bool (strict)"("DisabledEnum"=w1272) -> ()  [unwired: 2 in, 2 out]
        n1406 = property on="Analysis" class="Bool (strict)"("DisabledEnum"=w1272) -> ()  [unwired: 2 in, 2 out]
        n1407 = property on="Home" class="Bool (strict)"("DisabledEnum"=w1272) -> ()  [unwired: 2 in, 2 out]
        n1408 = property on="Report" class="Bool (strict)"("DisabledEnum"=w1272) -> ()  [unwired: 2 in, 2 out]
      }
    }
    n1409 = local read "Quit"() -> (w1200:bool)
    "Single" <- "Single - Graph"
  }
  n1410 = disable-structure shown="Disabled" {
    disable-tunnel: [w1552 _] -> w39
    disable-tunnel: _ -> [w1551 _]
    frame Disabled {
      n1411 = while {
        tunnel: w1551 -> [_]
        tunnel: [w1553] -> w1552
        tunnel: [w1554] -> _
        i -> [w1554]
        stop <- w1553 stop-if-true
        w1570 = u16 10 items=["1.0"=10, "1.5"=15, "2.0"=20] ("stop bits (10: 1 bit)")
        n1412 = Wait (ms)(milliseconds to wait=u32 10) -> ()  [unwired: 1 out]
        n1413 = call-poly "VISA Configure Serial Port"("VISA resource name"=refnum<visa-resource-name> "ASRL1::INSTR" ("COM PORT"), "timeout (10sec)"=u32 10, "baud rate (9600)"=u32 57600, "data bits (8)"=u16 8, "stop bits (10: 1 bit)"=w1570) -> ("VISA resource name out"=w1556:refnum<visa-resource-name>, "error out"=w1565:errorcluster)  [unwired: 9 in]
        n1414 = VISA Read(VISA resource name=w1556, byte count=u32 2 ("byte count (0)")) -> (read buffer=w1564:string)  [unwired: 1 in, 3 out]
        n1415 = String Subset(string=w1564, offset (0)=0, length (rest)=2 ("length (rest)")) -> (substring=w1563:string)
        n1416 = Match Pattern(string=w1563, regular expression="<>") -> (offset past match=w1560:i32)  [unwired: 1 in, 3 out]
        n1417 = Greater Or Equal?(x=w1560, y=0) -> (x >= y?=w1555:bool)
        n1418 = case shown="True" w1555 {
          tunnel: w1556 -> [_ w1574]
          tunnel: w1565 -> [_ w1573]
          frame False {
          }
          frame True {
            n1419 = VISA Read(VISA resource name=w1574, byte count=u32 32 ("byte count (0)"), error in (no error)=w1573) -> (read buffer=w1572:string)  [unwired: 3 out]
            n1420 = String Subset(string=w1572, offset (0)=0, length (rest)=8 ("length (rest)")) -> (substring=w1576:string)
            n1421 = String Subset(string=w1572, offset (0)=8, length (rest)=8 ("length (rest)")) -> (substring=w1577:string)
            n1422 = Decimal String To Number(string=w1577) -> (number=w1584:i32)  [unwired: 2 in, 1 out]
            n1423 = Decimal String To Number(string=w1576) -> (number=w1580:i32)  [unwired: 2 in, 1 out]
            n1424 = Divide(x=w1584, y=10000) -> ()  [unwired: 1 out]
            n1425 = Divide(x=w1580, y=1000000) -> ()  [unwired: 1 out]
          }
        }
        n1426 = local read "Quit"() -> (w1553:bool)
      }
    }
    frame Enabled {
    }
  }
  n1427 = while {
    shift-right: [w1599] -> w52
    shift-left: _ -> [w1590]
    shift-right: [w1598] -> w51
    shift-left: errorcluster {"status"=TRUE, "code"=0, "source"="Init"} ("error IO") -> [w1592]
    tunnel: [w1587] -> w42
    tunnel: [w1597] -> _
    i -> [w1597]
    stop <- w1587 stop-if-true
    n1428 = local read "Port 1a"() -> (w1593:bool)
    n1429 = local read "Port 3"() -> (w1594:bool)
    n1430 = local read "Com Port 1"() -> (w1591:refnum<visa-resource-name>)
    n1431 = Or(x=w1594, y=w1593) -> (x .or. y?=w1596:bool)
    n1432 = Unbundle(w1592) -> ("status"=→"Port 3":bool)  [unwired: 2 out]
    n1433 = Not Equal?(x=w1591, y=w1590) -> (x != y?=w1588:bool)
    n1434 = case shown="True" w1596 {
      frame False {
        w1602 = TRUE ("Visible")
        n1435 = property on="Port 1a" class="Bool (strict)"("Visible"=w1602) -> ()  [unwired: 2 in, 2 out]
        n1436 = property on="Port 3" class="Bool (strict)"("Visible"=w1602) -> ()  [unwired: 2 in, 2 out]
      }
      frame True {
        w1603 = TRUE ("Visible")
        n1437 = property on="Port 1a" class="Bool (strict)"("Visible"=w1603) -> ()  [unwired: 2 in, 2 out]
        n1438 = property on="Port 3" class="Bool (strict)"("Visible"=w1603) -> ()  [unwired: 2 in, 2 out]
      }
    }
    n1439 = Wait (ms)(milliseconds to wait=u32 40) -> ()  [unwired: 1 out]
    n1440 = case shown="True" w1588 {
      tunnel: [w1600 errorcluster {"status"=TRUE, "code"=0, "source"="Init"} ("error out")] -> w1589
      tunnel: w1592 -> [w1600 _]
      frame False {
      }
      frame True {
      }
    }
    n1441 = case shown="No Error" w1589 {
      selector: w1589 -> [w1611 w1638]
      tunnel: [w1605 w1642] -> w1599
      tunnel: [w1613 w1636] -> w1598
      tunnel: w1590 -> [w1612 w1640]
      frame No Error {
        n1442 = property class="Instr"(reference=w1612, error in=w1611) -> (reference out=w1609:refnum<visa-resource-name>, error out=w1610:errorcluster, "Serial Settings:Number of Bytes at Serial Port"=w1606:u32)
        n1443 = Greater?(x=w1606, y=u32 5) -> (0:w1604:bool)
        n1444 = Not(x=w1604) -> (.not. x?=→"Port 1a":bool)
        n1445 = while {
          tunnel: [w1631] -> w1613
          tunnel: [w1630] -> w1614
          tunnel: w1610 -> [w1629]
          tunnel: w1609 -> [w1628]
          stop <- TRUE stop-if-true
          n1446 = property class="Instr" props=["Serial Settings:Number of Bytes at Serial Port"](reference=w1628, error in=w1629) -> (reference out=w1633:refnum<visa-resource-name>, error out=w1632:errorcluster)  [unwired: 1 out]
          n1447 = VISA Read(VISA resource name=w1633, byte count=u32 50, error in (no error)=w1632) -> (VISA resource name out=w1630:refnum<visa-resource-name>, read buffer=w1615:string, error out=w1631:errorcluster)  [unwired: 1 out]
          "UNI READ" <- w1615
          n1448 = Spreadsheet String To Array(delimiter (Tab)=";", format string="", spreadsheet string=w1615, array type (2D Dbl)=dbl[] []) -> (array=w1625:dbl[])
          n1449 = Index Array(array=w1625) -> (element #1=→"LVDT MIN":dbl, element #2=→"LVDT MAX":dbl, element #3=→"LVDT Peak":dbl, element #4=→"pizo raw":dbl, element #5=→"Friction":dbl, element #6=→"cof 2":dbl)  [unwired: 6 in]
        }
        n1450 = VISA Flush I/O Buffer(VISA resource name=w1614) -> (VISA resource name out=w1605:refnum<visa-resource-name>)  [unwired: 2 in, 1 out]
      }
      frame Error {
        w1648 = u16 0 items=["None", "XON/XOFF", "RTS/CTS", "XON/XOFF & RTS/CTS", "DTR/DSR", "XON/XOFF & DTR/DSR"] ("flow control (0:none)  2")
        w1646 = u16 10 items=["1.0"=10, "1.5"=15, "2.0"=20] ("stop bits 2")
        w1644 = u16 0 items=["None", "Odd", "Even", "Mark", "Space"] ("parity 2")
        w1645 = u32 10000  # timeout (10sec)
        n1451 = VISA Close(VISA resource name=w1640, error in (no error)=w1638) -> (error out=w1641:errorcluster)
        n1452 = local write "Port 1a"(FALSE ("Port 1a")) -> ()
        n1453 = local read "Com Port 1"() -> (w1635:refnum<visa-resource-name>)
        n1454 = call <vilib>:"Clear Errors.vi"("error in (no error)"=w1641) -> ("error out"=w1639:errorcluster)  [unwired: 5 in, 1 out]
        n1455 = call-poly "VISA Configure Serial Port"("VISA resource name"=w1635, "timeout (10sec)"=w1645, "baud rate (9600)"=u32 250000 ("baud rate  2"), "data bits (8)"=u16 8 ("data bits  2"), "parity (0:none)"=w1644, "error in (no error)"=w1639, "stop bits (10: 1 bit)"=w1646, "flow control (0:none)"=w1648) -> ("VISA resource name out"=w1649:refnum<visa-resource-name>, "error out"=w1650:errorcluster)  [unwired: 6 in]
        n1456 = flat-sequence {
          tunnel: w1649 -> [w1652]
          tunnel: w1650 -> [w1651]
          tunnel: [w1652] -> w1642
          tunnel: [w1651] -> w1636
          frame #0 {
            n1457 = Wait (ms)(milliseconds to wait=u32 50) -> ()  [unwired: 1 out]
          }
        }
        "Residual Uno" <- ""
        "Port 1 Error" <- w1636
      }
    }
    n1458 = local read "Quit"() -> (w1587:bool)
    "Error Uno" <- w1592
  }
  n1459 = while {
    stop <- w1663 stop-if-true
    # "V0OLTAGE TO STROKE (peice vise calibration)"
    n1460 = local read "LVDT MIN"() -> (w1654:dbl)
    n1461 = Wait (ms)(milliseconds to wait=u32 10) -> ()  [unwired: 1 out]
    n1462 = local read "LVDT Peak"() -> (w1655:dbl)
